vi "MCL Single Read N.vi"(10 "handle":i32, 11 "axis":u32) -> (3 "function return":dbl)   [LabVIEW 2017, in "Madlib.lvlib"]
doc: "MADLIB_API double MCL_SingleReadN(unsigned int axis, int handle);"
uses:
  Madlib.lvlib
  Madlib.dll
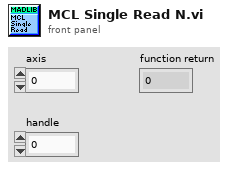
[diagram p1: front panel]
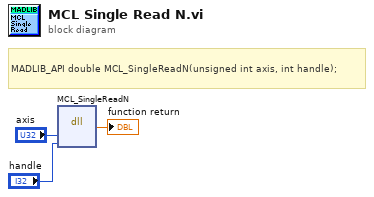
[diagram p0: block diagram]
diagram:
  # "MADLIB_API\tdouble\tMCL_SingleReadN(unsigned int axis, int handle);"
  n1 = dll-call lib="C:/Users/francesco/dev/pump-probe/Piezo/lvlib/Madlib.*" fn="MCL_SingleReadN"("axis"="axis", "handle"="handle") -> (→"function return":dbl)  [unwired: 5 in, 2 out]
